vi "Coder.vi"(1 "Запрос Вх":u8[](array[numeric])=[5, 0, 30] format="%02x") -> (0 "Запрос Вых":u8[](array[numeric])=[1, 5, 0, 30, 0, 0, 0, 0, 3] format="%02x")   [LabVIEW 2010]
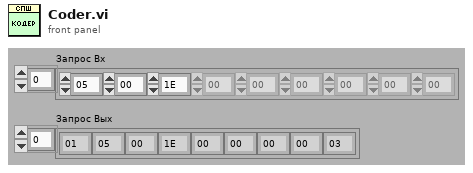
[diagram p1: front panel]
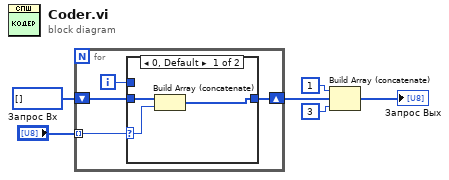
[diagram p0: block diagram]
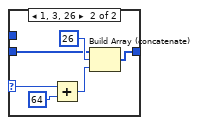
[diagram p2: hidden frame]
diagram:
  n1 = for {
    tunnel: "Запрос Вх" -> [w10] mode=indexing
    shift-right: [w8] -> w4
    shift-left: u8[] [] ("appended array") -> [w9]
    i -> [w7]
    n2 = case shown="0, Default" w10 {
      selector: w10 -> [w12 w19]
      tunnel: w9 -> [w13 w15]
      tunnel: [w11 w14] -> w8
      tunnel: w7 -> [_ _]
      frame 0, Default {
        n3 = Build Array (concatenate)(w13, w12) -> (w11:u8[])
      }
      frame 1, 3, 26 {
        n4 = Add(x=w19, y=u8 64 ("Numeric")) -> (x+y=w16:u8)
        n5 = Build Array (concatenate)(w15, u8 26 ("Numeric"), w16) -> (w14:u8[])
      }
    }
  }
  n6 = Build Array (concatenate)(u8 1 ("Numeric"), w4, u8 3 ("Numeric")) -> (→"Запрос Вых":u8[])
